vi "Handle getAll.vi"(8 "error in (no error)":errorcluster, 11 "Sequence Experiment":refnum<class "SMO.Control Experiment.lvclass">) -> (0 "error out":errorcluster, 2 "getAll":variant, 3 "Sequence Experiment out":refnum<class "SMO.Control Experiment.lvclass">)   [LabVIEW 2019, in "SMO.Control Experiment.lvclass"]
uses:
  SMO.Control Experiment.lvclass
  <userlib>/LevyLab/Instrument Framework/SMOs/Instrument/Instrument.lvclass
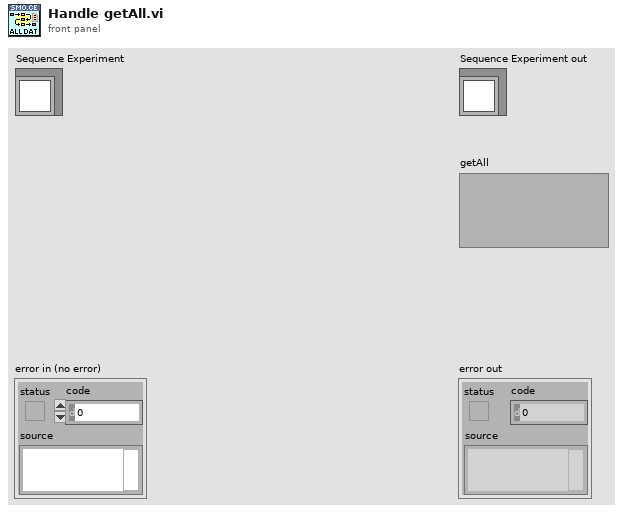
[diagram p1: front panel]
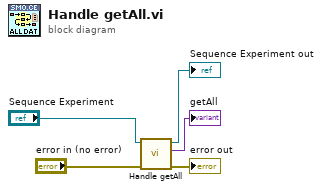
[diagram p0: block diagram]
diagram:
  n1 = call-parent "Handle getAll.vi"("error in (no error)"="error in (no error)", "Instrument in"="Sequence Experiment") -> ("error out"=→"error out":errorcluster, "getAll"=→"getAll":variant, "Instrument out"=→"Sequence Experiment out":refnum<class "SMO.Control Experiment.lvclass">)  [unwired: 7 in]
